vi "Generate Error Event.vi"(8 "error in (no error)":errorcluster, 10 "Error":errorcluster, 11 "GIS Printer in":refnum<class "GIS Printer.lvclass">) -> (0 "error out":errorcluster, 3 "GIS Printer out":refnum<class "GIS Printer.lvclass">)   [LabVIEW 2022 SP3, in "GIS Printer.lvclass"]
uses:
  GIS Printer.lvclass
  TopLevel/Typedefs/Error Data Cluster.ctl
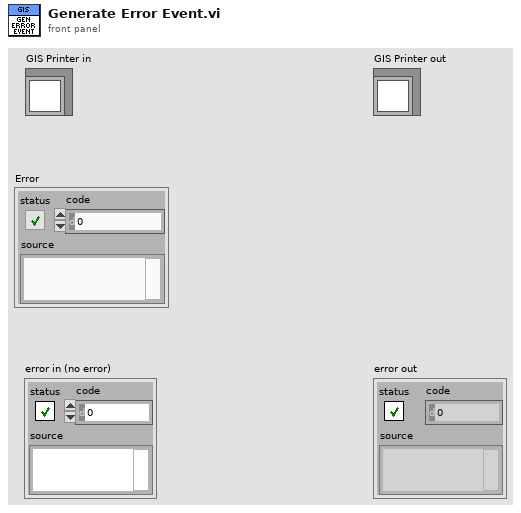
[diagram p1: front panel]
types:
  T1 = typedef "Error Data Cluster.ctl" = cluster{"TimeStamp":timestamp, "Error":errorcluster}
  T2 = typedef "GIS Printer.lvclass/UserEvents.ctl" = cluster{"API Incoming Event":refnum<user-event>, "API Executed Event":refnum<user-event>, "API Return Event":refnum<user-event>, "Status Changed Event":refnum<user-event>, "Abort":refnum<user-event>, "stop process":refnum<user-event>, "GISPollStatus":refnum<user-event>, "GISHeadStatus":refnum<user-event>, "Error Event":refnum<user-event>}
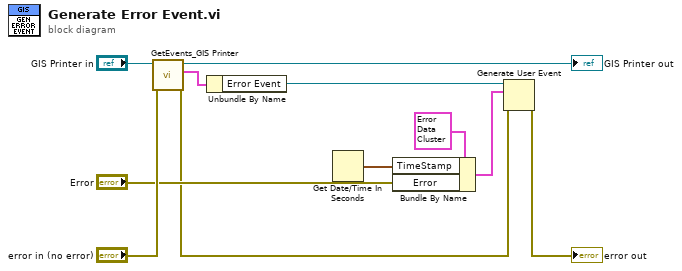
[diagram p0: block diagram]
diagram:
  n1 = call-dynamic "GetEvents_GIS Printer.vi"("error in (no error)"="error in (no error)", "TopLevel in"="GIS Printer in") -> ("error out"=w2:errorcluster, "UserEvents"=w9:T2, "TopLevel out"=→"GIS Printer out":refnum<class "GIS Printer.lvclass">)  [unwired: 7 in]
  n2 = Unbundle By Name(w9) -> ("Error Event"=w3:refnum<user-event>)
  n3 = Get Date/Time In Seconds() -> (seconds since 1Jan1904=w7:timestamp)
  n4 = Bundle By Name(cluster=T1 {"TimeStamp"=timestamp(0 s since 1904-01-01), "Error"={"status"=FALSE, "code"=0, "source"=""}} ("event data"), "TimeStamp"=w7, "Error"="Error") -> (w6:T1)
  n5 = Generate User Event(user event=w3, event data cluster=w6, error in=w2) -> (error out=→"error out":errorcluster)  [unwired: 1 in, 1 out]
